vi "Set70dbAtten2.vi"(8 "error in (no error)":errorcluster, 11 "Attenuation (dB)":i32=70 min=0 max=70 step=10) -> (0 "error out":errorcluster, 2 "Verfied":bool, 3 "Active Attenuators":bool[](array[boolean])=[FALSE, TRUE, TRUE, TRUE])   [LabVIEW 2012]
doc: "Opens channel for specified ID"
panel:
  out "Closed Switches - Inactive Atten":string
  out "Open Switches - Active Atten":string="7141,7142,7143"
  # "70 dB Attenuator Switch"
  # "10 dB"
  # "20 dB"
  # "40 dB"
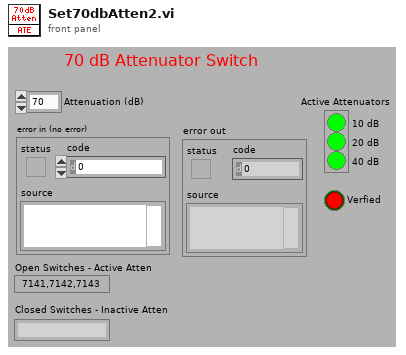
[diagram p1: front panel]
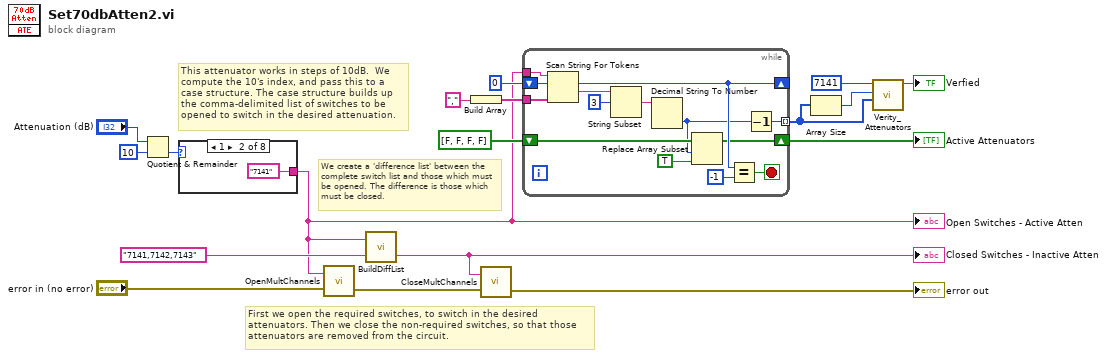
[diagram p0: block diagram]
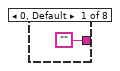
[diagram p2: hidden frame]
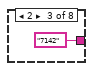
[diagram p3: hidden frame]
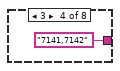
[diagram p4: hidden frame]
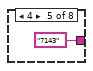
[diagram p5: hidden frame]
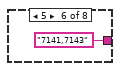
[diagram p6: hidden frame]
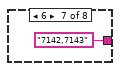
[diagram p7: hidden frame]
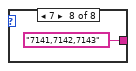
[diagram p8: hidden frame]
diagram:
  # "First we open the required switches, to switch in the desired attenuators. Then we close the non-required switches, so that those attenuators are removed from the circuit."
  # "We create a 'difference list' between the complete switch list and those which must be opened. The difference is those which must be closed."
  # "This attenuator works in steps of 10dB.  We compute the 10's index, and pass this to a case structure. The case structure builds up the comma-delimited list of switches to be opened to switch in the desired attenuation."
  n1 = Quotient & Remainder(x="Attenuation (dB)", y=10) -> (floor(x/y)=w12:i32)  [unwired: 1 out]
  n2 = case shown="1" w12 {
    tunnel: ["" "7141" "7142" "7141,7142" "7143" "7141,7143" "7142,7143" "7141,7142,7143"] -> w6
    frame 0, Default {
    }
    frame 1 {
    }
    frame 2 {
    }
    frame 3 {
    }
    frame 4 {
    }
    frame 5 {
    }
    frame 6 {
    }
    frame 7 {
    }
  }
  "Open Switches - Active Atten" <- w6
  n3 = call "OpenMultChannels.vi"("error in (no error)"="error in (no error)", "Channels to be opened"=w6) -> ("error out"=w16:errorcluster)  [unwired: 1 in]
  n4 = call "BuildDiffList.vi"("Reference list"="7141,7142,7143", "Input list"=w6) -> ("Difference list"=w7:string)  [unwired: 1 in]
  "Closed Switches - Inactive Atten" <- w7
  n5 = Build Array(",") -> (w10:string[])
  n6 = call "CloseMultChannels.vi"("error in (no error)"=w16, "Channels to be closed"=w7) -> ("error out"=→"error out":errorcluster)  [unwired: 1 in]
  n7 = while {
    tunnel: w10 -> [w38]
    shift-right: [w36] -> _
    shift-left: 0 ("offset") -> [w37]
    tunnel: w6 -> [w40]
    shift-right: [w29] -> w5
    shift-left: bool[] [FALSE, FALSE, FALSE, FALSE] -> [w32]
    tunnel: [w27] -> w2 mode=indexing
    stop <- w30 stop-if-true
    n8 = Scan String For Tokens(6:w38, 8:w37, 9:w40) -> (1:w35:string, 2:w36:i32)  [unwired: 3 in, 2 out]
    n9 = String Subset(string=w35, offset (0)=3) -> (substring=w33:string)  [unwired: 1 in]
    n10 = Decimal String To Number(string=w33) -> (number=w28:i32)  [unwired: 2 in, 1 out]
    n11 = Replace Array Subset(array=w32, new element=TRUE ("new element/subarray"), index=w28) -> (w29:bool[])
    n12 = Equal?(x=w36, y=-1) -> (x = y?=w30:bool)
    n13 = Decrement(x=w28) -> (x-1=w27:i32)
  }
  "Active Attenuators" <- w5
  n14 = Array Size(array=w2) -> (size(s)=w1:i32)
  n15 = call "Verity_Attenuators.vi"("Switches"=w2, "nSwitches"=w1, "Base Switch ID"=7141) -> ("Verfied"=→"Verfied":bool)  [unwired: 8 in]
